vi "Periodic Tasks.vi"(8 "error in":errorcluster) -> ()   [LabVIEW 2015]
doc: "This VI runs in parallel to other tasks. It can contain as many user-defined periodic loops as you need. These can carry out PID or other sorts of timed response."
uses:
  <vilib>/Rock Robotics/WPI/Utilities/WPI_GetSetVariantRefNum.vi
  <vilib>/Rock Robotics/Network Tables/NT Write Boolean.vi
  <vilib>/Rock Robotics/Network Tables/NT Write Number.vi
panel:
  out "Gyro":dbl
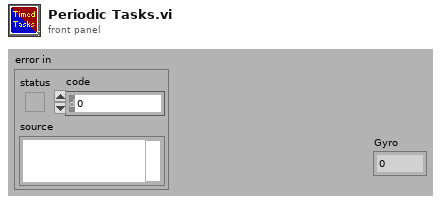
[diagram p1: front panel]
types:
  T1 = typedef "WPI_JoystickDevRef.ctl" = cluster{"Device":T2}
  T2 = typedef "WPI_JoystickDeviceEnum.ctl" = enum16{"USB 0", "USB 1", "USB 2", "USB 3", "USB 4", "USB 5"}
  T3 = typedef "WPI_RobotDriveDevRef.ctl" = cluster{"DevStatus":errorcluster, "Motors[]":T4[], "Square Inputs":bool, "Max Output":dbl}
  T4 = typedef "WPI_MotorControlDeviceRef.ctl" = cluster{"DeviceStatus":errorcluster, "Type":T5, "PWM":cluster{"PWM Channel":T6, "DeadBand":T7}, "CAN":cluster{"Device Number":u8, "Control Mode":T8, "Semaphore":T9, "Max Vout":dbl, "TalonSRX Control Mode":T10}, "Invert":bool}
  T5 = typedef "WPI_MotorControlType.ctl" = enum16{"PWM", "CAN", "CANTalonSRX"}
  T6 = typedef "FPGA_DIOPWMChannel.ctl" = enum8{"PWM 0", "PWM 1", "PWM 2", "PWM 3", "PWM 4", "PWM 5", "PWM 6", "PWM 7", "PWM 8", "PWM 9", "PWM MXP 0", "PWM MXP 1", "PWM MXP 2", "PWM MXP 3", "PWM MXP 4", "PWM MXP 5", "PWM MXP 6", "PWM MXP 7", "PWM MXP 8", "PWM MXP 9", "Invalid"}
  T7 = typedef "WPI_PWMDeadband.ctl" = cluster{"Name":string, "maxPositivePwm":i32, "minPositivePwm":i32, "centerPwm":i32, "maxNegativePwm":i32, "minNegativePwm":i32, "angularRange":u16}
  T8 = typedef "WPI_CANJaguar_ControlMode.ctl" = enum8{"Percent VBus", "Current", "Speed", "Position", "Voltage"}
  T9 = typedef "Semaphore RefNum" = refnum<k1>
  T10 = typedef "WPI_CANTalonSRX_APIControlMode.ctl" = enum8{"Percent VBus", "Speed", "Position", "Slave", "Unchanged / Invalid", "Voltage Compensation", "Current", "Motion Profile"}
  T11 = cluster{"JoystickDevRef":T1, "RobotDriveDevRef":T3}
  T12 = typedef "WPI_CompressorDevRef.ctl" = cluster{"DevStatus":errorcluster, "Pneumatics Control Module":u8}
  T13 = typedef "WPI_AccelerometerDevRef.ctl" = cluster{"DevStatus":errorcluster, "Scaling":T14, "Analog Channels":T15, "I2C Bus":T17, "SPI Bus":T18, "Accel Range":T19, "ADXL Axes":T20, "Handle":i32, "Device Address":u8, "Accel Type":enum16{"Analog", "ADXL345 I2C", "ADXL345 SPI", "Internal", "ADXL362 SPI"}}
  T14 = typedef "WPI_AccelerometerScaling.ctl" = cluster{"Gain (VoltsPerG)":dbl, "Center Voltage":dbl}
  T15 = typedef "WPI_AccelerometerAnalogChannels.ctl" = cluster{"X-Axis":T16, "Y-Axis":T16, "Z-Axis":T16}
  T16 = typedef "FPGA_AIChannel.ctl" = enum8{"AI 0", "AI 1", "AI 2", "AI 3", "AI MXP 0", "AI MXP 1", "AI MXP 2", "AI MXP 3", "Invalid"}
  T17 = typedef "i2c_bus.ctl" = enum16{"I2C On-Board", "I2C MXP", "Invalid"}
  T18 = typedef "spi_bus.ctl" = enum16{"SPI On-Board, CS0", "SPI On-Board, CS1", "SPI On-Board, CS2", "SPI On-Board, CS3", "SPI MXP", "Invalid"}
  T19 = typedef "ADXL345 Range.ctl" = u8
  T20 = typedef "WPI_AccelerometerADXL345 Axes.ctl" = cluster{"X-Axis":bool, "Y-Axis":bool, "Z-Axis":bool}
  T21 = cluster{"X-Axis":dbl, "Y-Axis":dbl, "Z-Axis":dbl}
  T22 = typedef "WPI_GyroDevRef.ctl" = cluster{"DevStatus":errorcluster, "Analog Channel":T16, "Offset":dbl, "Gain (VoltsPerDegree/Second)":dbl, "Gyro Type":enum16{"Analog", "XRS450"}, "Handle":i32, "SPI Bus":T18, "Device Found":bool, "Sample Rate":dbl, "Calibrate On Open":bool}
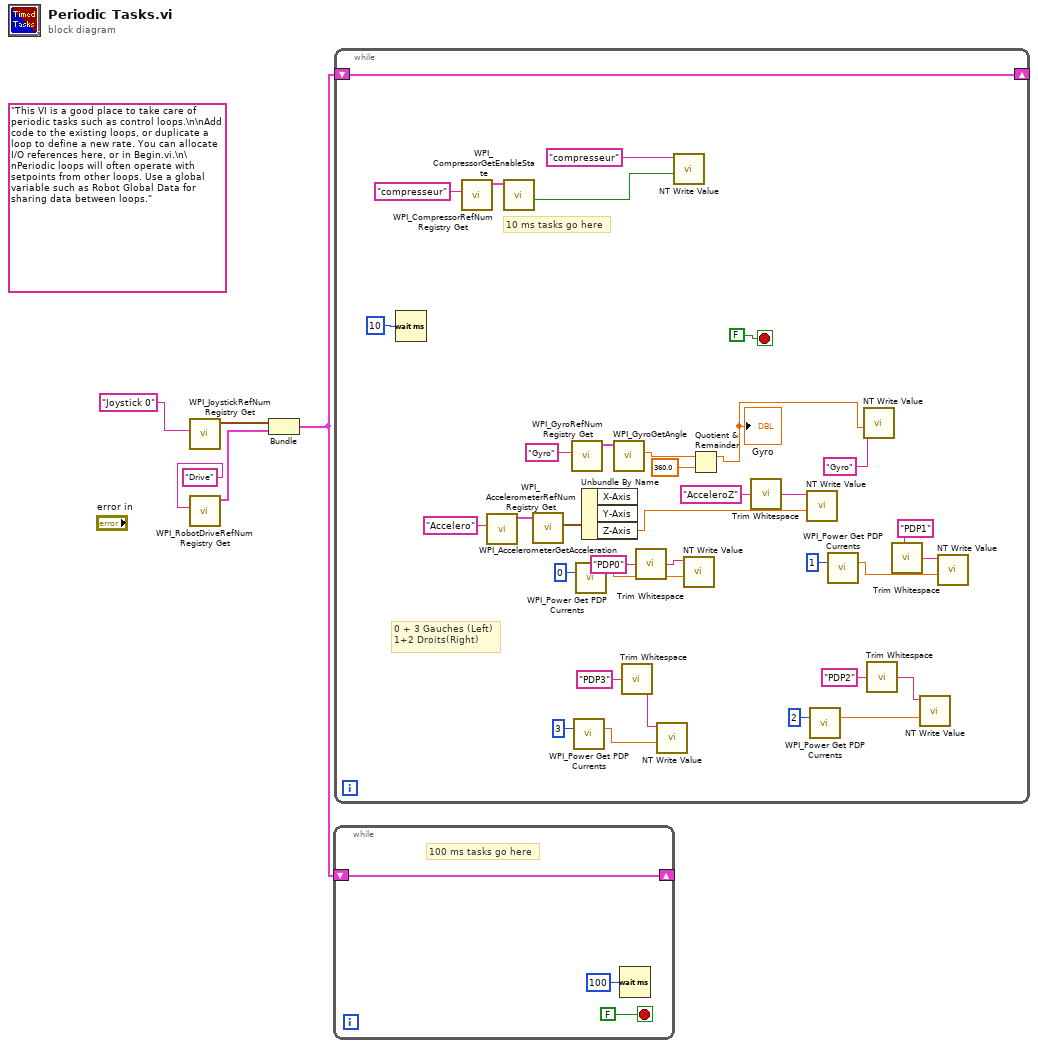
[diagram p0: block diagram]
diagram:
  (unwired) "This VI is a good place to take care of periodic tasks such as control loops.\n\nAdd code to the existing loops, or duplicate a loop to define a new rate. You can allocate I/O references here, or in Begin.vi.\n\nPeriodic loops will often operate with setpoints from other loops. Use a global variable such as Robot Global Data for sharing data between loops."
  n1 = call <vilib>:"WPI_JoystickRefNum Registry Get.vi"("refnum name"="Joystick 0") -> ("JoystickDevRef"=w3:T1)  [unwired: 1 in, 9 out]
  n2 = call <vilib>:"WPI_RobotDriveRefNum Registry Get.vi"("refnum name"="Drive") -> ("RobotDriveDevRef"=w2:T3)  [unwired: 1 in, 9 out]
  n3 = Bundle("JoystickDevRef"=w3, "RobotDriveDevRef"=w2) -> (w1:T11)  [unwired: 1 out]
  n4 = while {
    shift-right: [w6] -> _
    shift-left: w1 -> [w6]
    stop <- FALSE stop-if-true
    # "100 ms tasks go here"
    n5 = Wait (ms)(milliseconds to wait=u32 100) -> ()  [unwired: 1 out]
  }
  n6 = while {
    shift-right: [w41] -> _
    shift-left: w1 -> [w41]
    stop <- FALSE stop-if-true
    # "0 + 3 Gauches (Left)\n1+2 Droits(Right)"
    # "10 ms tasks go here"
    n7 = Wait (ms)(milliseconds to wait=u32 10) -> ()  [unwired: 1 out]
    n8 = call <vilib>:"WPI_CompressorRefNum Registry Get.vi"("refnum name"="compresseur") -> ("CompressorDevRef"=w40:T12)  [unwired: 9 in, 1 out]
    n9 = call <vilib>:"WPI_AccelerometerRefNum Registry Get.vi"("refnum name"="Accelero") -> ("AccelerometerDevRef"=w33:T13)  [unwired: 9 in, 1 out]
    n10 = call <vilib>:"WPI_CompressorGetEnableState.vi"("CompressorDevRef"=w40) -> ("Compressor Running"=w9:bool)  [unwired: 7 in, 3 out]
    n11 = call <vilib>:"WPI_AccelerometerGetAcceleration.vi"("AccelerometerDevRef"=w33) -> ("Accelerations"=w31:T21)  [unwired: 8 in, 2 out]
    n12 = call <vilib>:"WPI_GyroRefNum Registry Get.vi"("refnum name"="Gyro") -> ("GyroDevRef"=w37:T22)  [unwired: 9 in, 1 out]
    n13 = call <vilib>:"WPI_Power Get PDP Currents.vi"("PDP Channel"=3) -> ("current (A)"=w24:dbl)  [unwired: 12 in, 2 out]
    n14 = call <vilib>:"WPI_Power Get PDP Currents.vi"("PDP Channel"=0) -> ("current (A)"=w23:dbl)  [unwired: 12 in, 2 out]
    n15 = Unbundle By Name(w31) -> ("Z-Axis"=w12:dbl)  [unwired: 2 out]
    n16 = call <vilib>:"WPI_GyroGetAngle.vi"("GyroDevRef"=w37) -> ("Angle"=w35:dbl)  [unwired: 6 in, 4 out]
    n17 = call <vilib>:"Trim Whitespace.vi"("string"="PDP3") -> ("trimmed string"=w20:string)  [unwired: 1 in]
    n18 = call <vilib>:"Trim Whitespace.vi"("string"="PDP0") -> ("trimmed string"=w18:string)  [unwired: 1 in]
    n19 = call-poly <vilib>:"NT Write Value.vi"("Numeric"=w24, "Name"=w20) -> ()  [unwired: 9 in, 1 out]
    n20 = call-poly <vilib>:"NT Write Value.vi"("Boolean"=w9, "Name"="compresseur") -> ()  [unwired: 9 in, 1 out]
    n21 = call-poly <vilib>:"NT Write Value.vi"("Numeric"=w23, "Name"=w18) -> ()  [unwired: 9 in, 1 out]
    n22 = Quotient & Remainder(x=w35, y=360.0) -> (x-y*floor(x/y)=w11:dbl)  [unwired: 1 out]
    "Gyro" <- w11
    n23 = call <vilib>:"Trim Whitespace.vi"("string"="AcceleroZ") -> ("trimmed string"=w29:string)  [unwired: 1 in]
    n24 = call-poly <vilib>:"NT Write Value.vi"("Numeric"=w12, "Name"=w29) -> ()  [unwired: 9 in, 1 out]
    n25 = call <vilib>:"WPI_Power Get PDP Currents.vi"("PDP Channel"=2) -> ("current (A)"=w21:dbl)  [unwired: 12 in, 2 out]
    n26 = call <vilib>:"WPI_Power Get PDP Currents.vi"("PDP Channel"=1) -> ("current (A)"=w22:dbl)  [unwired: 12 in, 2 out]
    n27 = call-poly <vilib>:"NT Write Value.vi"("Numeric"=w11, "Name"="Gyro") -> ()  [unwired: 9 in, 1 out]
    n28 = call <vilib>:"Trim Whitespace.vi"("string"="PDP2") -> ("trimmed string"=w14:string)  [unwired: 1 in]
    n29 = call <vilib>:"Trim Whitespace.vi"("string"="PDP1") -> ("trimmed string"=w16:string)  [unwired: 1 in]
    n30 = call-poly <vilib>:"NT Write Value.vi"("Numeric"=w21, "Name"=w14) -> ()  [unwired: 9 in, 1 out]
    n31 = call-poly <vilib>:"NT Write Value.vi"("Numeric"=w22, "Name"=w16) -> ()  [unwired: 9 in, 1 out]
  }
